vi "Update Log Status Values.vi"(1 "RT Data in":T1={"Device Ref"=18446744073709551615, "Waveforms"=[], "Channels"={"Command Chan Refs"=[], "Command Data Refs"=[], "Command Values"=[], "Status Chan Refs"=[], "Status Data Refs"=[], "Status Values"=[], "System Time"={"System Time"=timestamp(0 s since 1904-01-01), "Data Reference"=0, "Absolute Time Channel Data Ref"=0, "Get Date-Time Channel Data Ref"=0}, "Trigger Chan Refs"=[], "Trigger Data Refs"=[], "Trigger Values"=[]}, "Waveform Logs"=[], "Communication"={"Async Status"=refnum, "Wfm Comm Properties"={"WPL"={"Custom Queue Size"=1, "Use Custom Queue Size?"=FALSE}}, "Shutdown Event"=refnum, "Trigger Event"=refnum, "New File Event"=refnum, "Log Queues"=[], "Async VI Ref"=refnum}, "error"={"status"=FALSE, "code"=0, "source"=""}} {"Device Ref" format="%.0x"; "Channels"."Trigger Data Refs"."Data Reference" format="%.0x"; "Channels"."Trigger Chan Refs" format="%.0x"; "Channels"."System Time"."Get Date-Time Channel Data Ref" format="%.0x"; "Channels"."System Time"."Absolute Time Channel Data Ref" format="%.0x"; "Channels"."System Time"."Channel Data Reference" format="%.0x"; "Channels"."Status Data Refs"."Data Reference" format="%.0x"; "Channels"."Command Data Refs"."Data Reference" format="%.0x"; "Channels"."Status Chan Refs" format="%.0x"; "Channels"."Command Chan Refs" format="%.0x"; "Waveforms"."Waveform Ref in" format="%.0x"; "Waveform Logs"."Node ID" format="%.0x"; "Waveform Logs"."TDMS Error Code"."Data Ref" format="%.0x"; "Waveform Logs"."Missed Samples"."Data Ref" format="%.0x"; "Waveform Logs"."File Status"."Data Ref" format="%.0x"; "Waveform Logs"."Start New File"."Data Ref" format="%.0x"; "Waveform Logs"."Logging Enabled"."Data Ref" format="%.0x"; "Waveform Logs"."Stop Trigger"."Node Data Ref" format="%.0x"; "Waveform Logs"."Stop Trigger"."Node ID" format="%.0x"; "Waveform Logs"."Start Trigger"."Node Data Ref" format="%.0x"; "Waveform Logs"."Start Trigger"."Node ID" format="%.0x"}) -> (0 "RT Data out":T1={"Device Ref"=18446744073709551615, "Waveforms"=[], "Channels"={"Command Chan Refs"=[], "Command Data Refs"=[], "Command Values"=[], "Status Chan Refs"=[], "Status Data Refs"=[], "Status Values"=[], "System Time"={"System Time"=timestamp(0 s since 1904-01-01), "Data Reference"=0, "Absolute Time Channel Data Ref"=0, "Get Date-Time Channel Data Ref"=0}, "Trigger Chan Refs"=[], "Trigger Data Refs"=[], "Trigger Values"=[]}, "Waveform Logs"=[], "Communication"={"Async Status"=refnum, "Wfm Comm Properties"={"WPL"={"Custom Queue Size"=1, "Use Custom Queue Size?"=FALSE}}, "Shutdown Event"=refnum, "Trigger Event"=refnum, "New File Event"=refnum, "Log Queues"=[], "Async VI Ref"=refnum}, "error"={"status"=FALSE, "code"=0, "source"=""}} {"Device Ref" format="%.0x"; "Channels"."Trigger Data Refs"."Data Reference" format="%.0x"; "Channels"."Trigger Chan Refs" format="%.0x"; "Channels"."System Time"."Get Date-Time Channel Data Ref" format="%.0x"; "Channels"."System Time"."Absolute Time Channel Data Ref" format="%.0x"; "Channels"."System Time"."Channel Data Reference" format="%.0x"; "Channels"."Status Data Refs"."Data Reference" format="%.0x"; "Channels"."Command Data Refs"."Data Reference" format="%.0x"; "Channels"."Status Chan Refs" format="%.0x"; "Channels"."Command Chan Refs" format="%.0x"; "Waveforms"."Waveform Ref in" format="%.0x"; "Waveform Logs"."Node ID" format="%.0x"; "Waveform Logs"."TDMS Error Code"."Data Ref" format="%.0x"; "Waveform Logs"."Missed Samples"."Data Ref" format="%.0x"; "Waveform Logs"."File Status"."Data Ref" format="%.0x"; "Waveform Logs"."Start New File"."Data Ref" format="%.0x"; "Waveform Logs"."Logging Enabled"."Data Ref" format="%.0x"; "Waveform Logs"."Stop Trigger"."Node Data Ref" format="%.0x"; "Waveform Logs"."Stop Trigger"."Node ID" format="%.0x"; "Waveform Logs"."Start Trigger"."Node Data Ref" format="%.0x"; "Waveform Logs"."Start Trigger"."Node ID" format="%.0x"})   [LabVIEW 2015, in "Waveform Data Logger Engine.lvlib"]
uses:
  Waveform Data Logger Engine.lvlib
  Types/RT Data.ctl
  <vilib>/NI Veristand/Custom Device API/Custom Device Item Ref.ctl
  Types/Inline Waveform Info.ctl
  <vilib>/NI Veristand/Custom Device API/Waveform Data Reference.ctl
  Classes/Waveforms/Waveform Receive/Associated Log.ctl
  <vilib>/NI Veristand/Custom Device API/Custom Device Waveform DataType.ctl
  Types/Channels.ctl
  <vilib>/NI Veristand/Custom Device API/Block Data Reference.ctl
  <vilib>/NI Veristand/Custom Device API/Data Reference.ctl
  Types/System Time.ctl
  Types/Inline Waveform Log Info.ctl
  Classes/Log File Specifications/Waveform TDMS Log File Specification/Waveform TDMS Log File Specification.lvclass
  Classes/Triggers/Trigger/Trigger.lvclass
  Types/Inline Log Waveform.ctl
  Types/Trigger Settings.ctl
  Types/Log Status.ctl
  Types/Channel.ctl
  Types/Communication.ctl
  Types/Async Status.ctl
  Types/Async State.ctl
  <vilib>/NI Veristand/Custom Device Waveform API/Communication Properties.ctl
  Types/Trigger Event Data.ctl
  Types/Trigger Received.ctl
  Types/New File Event Data.ctl
  Types/Log Queues.ctl
  <vilib>/NI Veristand/Custom Device API/Custom Device API.lvlib
  Classes/Waveforms/Waveform Receive/Waveform Receive.lvclass
  <vilib>/NI Veristand/Custom Device Waveform API/NI_VS Custom Device Waveform API.lvlib
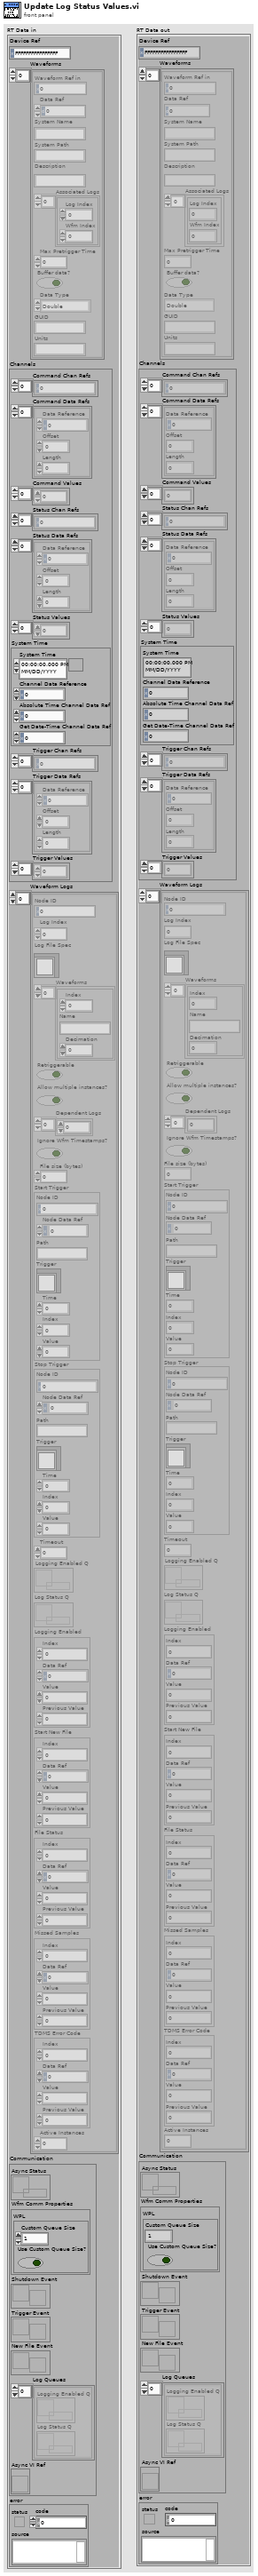
[diagram p1: front panel]
types:
  T1 = typedef "Waveform Data Logger Engine.lvlib/RT Data.ctl" = cluster{"Device Ref":T2, "Waveforms":T3[], "Channels":T7, "Waveform Logs":T11[], "Communication":T15, "error":errorcluster}
  T2 = typedef "Custom Device API.lvlib/Custom Device Item Ref.ctl" = u64
  T3 = typedef "Waveform Data Logger Engine.lvlib/Inline Waveform Info.ctl" = cluster{"Waveform Ref in":T2, "Data Ref":T4, "System Name":string, "System Path":string, "Description":string, "Associated Logs":T5[], "Max Pretrigger Time":dbl, "Buffer data?":bool, "Data Type":T6, "GUID":string, "Units":string}
  T4 = typedef "Custom Device API.lvlib/Waveform Data Reference.ctl" = i32
  T5 = typedef "Waveform Receive.lvclass/Associated Log.ctl" = cluster{"Log Index":i32, "Wfm Index":i32}
  T6 = typedef "Custom Device API.lvlib/Custom Device Waveform DataType.ctl" = enum16{"Double", "Complex Double"}
  T7 = typedef "Waveform Data Logger Engine.lvlib/Channels.ctl" = cluster{"Command Chan Refs":T2[], "Command Data Refs":T8[], "Command Values":dbl[], "Status Chan Refs":T2[], "Status Data Refs":T8[], "Status Values":dbl[], "System Time":T10, "Trigger Chan Refs":T2[], "Trigger Data Refs":T8[], "Trigger Values":dbl[]}
  T8 = typedef "Custom Device API.lvlib/Block Data Reference.ctl" = cluster{"Data Reference":T9, "Offset":u64, "Length":u64}
  T9 = typedef "Custom Device API.lvlib/Data Reference.ctl" = i32
  T10 = typedef "Waveform Data Logger Engine.lvlib/System Time.ctl" = cluster{"System Time":timestamp, "Data Reference":T9, "Absolute Time Channel Data Ref":T9, "Get Date-Time Channel Data Ref":T9}
  T11 = typedef "Waveform Data Logger Engine.lvlib/Inline Waveform Log Info.ctl" = cluster{"Node ID":T2, "Log Index":i32, "Log File Spec":refnum<class "Waveform TDMS Log File Specification.lvclass">, "Waveforms":T12[], "Retriggerable":bool, "Allow multiple instances?":bool, "Dependent Logs":i32[], "Ignore Wfm Timestamps?":bool, "File size (bytes)":i64, "Start Trigger":T13, "Stop Trigger":T13, "Timeout":dbl, "Logging Enabled Q":refnum<queue>, "Log Status Q":refnum<queue>, "Logging Enabled":T14, "Start New File":T14, "File Status":T14, "Missed Samples":T14, "TDMS Error Code":T14, "Active Instances":i32}
  T12 = typedef "Waveform Data Logger Engine.lvlib/Inline Log Waveform.ctl" = cluster{"Index":i32, "Name":string, "Decimation":u32}
  T13 = typedef "Waveform Data Logger Engine.lvlib/Trigger Settings.ctl" = cluster{"Node ID":T2, "Node Data Ref":i32, "Path":string, "Trigger":refnum<class "Trigger.lvclass">, "Time":dbl, "Index":i32, "Value":dbl}
  T14 = typedef "Waveform Data Logger Engine.lvlib/Channel.ctl" = cluster{"Index":i32, "Data Ref":T9, "Value":dbl, "Previous Value":dbl}
  T15 = typedef "Waveform Data Logger Engine.lvlib/Communication.ctl" = cluster{"Async Status":refnum<queue>, "Wfm Comm Properties":T16, "Shutdown Event":refnum<user-event>, "Trigger Event":refnum<user-event>, "New File Event":refnum<user-event>, "Log Queues":T17[], "Async VI Ref":refnum<vi>}
  T16 = typedef "NI_VS Custom Device Waveform API.lvlib/Communication Properties.ctl" = cluster{"WPL":cluster{"Custom Queue Size":i32, "Use Custom Queue Size?":bool}}
  T17 = typedef "Waveform Data Logger Engine.lvlib/Log Queues.ctl" = cluster{"Logging Enabled Q":refnum<queue>, "Log Status Q":refnum<queue>}
  T18 = typedef "Waveform Data Logger Engine.lvlib/Log Status.ctl" = cluster{"Open Instances":i32, "Active Instances":i32, "Missed Samples":u64, "Error Code":i32}
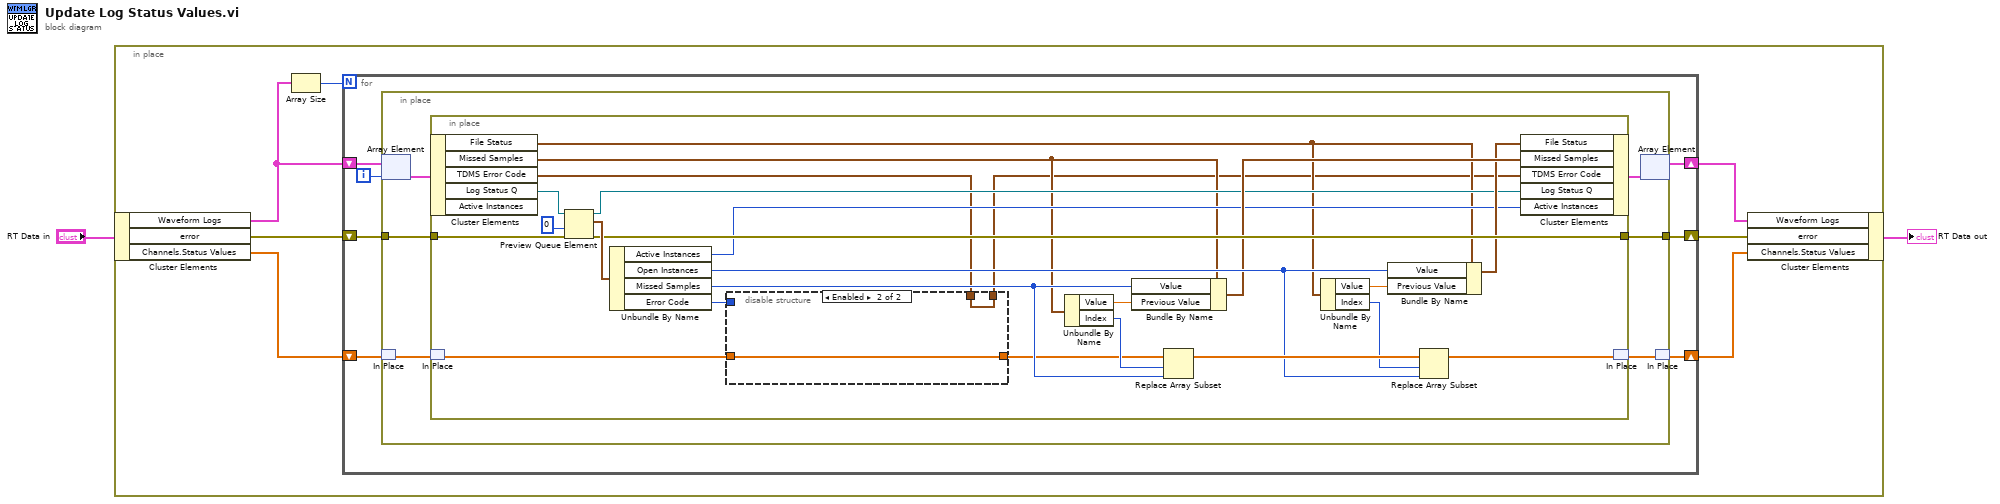
[diagram p0: block diagram]
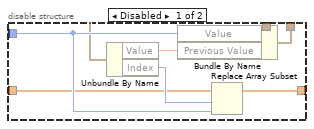
[diagram p2: hidden frame]
diagram:
  n1 = in-place {
    n2 = in-place-cluster #1("RT Data in") -> ("Waveform Logs"=w7:T11[], "error"=w9:errorcluster, "Channels.Status Values"=w4:dbl[])
    n3 = Array Size(array=w7) -> (size(s)=w8:i32)
    n4 = for {
      N: w8 -> [_]
      shift-right: [w12] -> w6
      shift-left: w9 -> [w16]
      shift-right: [w13] -> w5
      shift-left: w7 -> [w14]
      shift-right: [w10] -> w3
      shift-left: w4 -> [w11]
      i -> [w15]
      n5 = in-place {
        in-place-border: w16 -> [w22]
        in-place-border: [w21] -> w12
        n6 = in-place-array #2(w14, w15) -> (w18:T11)
        n7 = in-place-match #3(w11) -> (w20:dbl[])
        n8 = in-place {
          in-place-border: w22 -> [w44]
          in-place-border: [w43] -> w21
          n9 = in-place-cluster #4(w18) -> ("File Status"=w27:T14, "Missed Samples"=w30:T14, "TDMS Error Code"=w23:T14, "Log Status Q"=w34:refnum<queue>)  [unwired: 1 out]
          n10 = in-place-match #5(w20) -> (w41:dbl[])
          n11 = Preview Queue Element(queue=w34, timeout in ms (-1)=0, error in (no error)=w44) -> (queue out=w33:refnum<queue>, element=w45:T18, error out=w43:errorcluster)  [unwired: 1 out]
          n12 = Unbundle By Name(w45) -> ("Active Instances"=w32:i32, "Open Instances"=w39:i32, "Missed Samples"=w38:u64, "Error Code"=w26:i32)
          n13 = disable-structure shown="Enabled" {
            disable-tunnel: w26 -> [w51 _]
            disable-tunnel: [w50 w55] -> w25
            disable-tunnel: w23 -> [w49 w55]
            disable-tunnel: w41 -> [w48 w54]
            disable-tunnel: [w47 w54] -> w24
            frame Disabled {
              n14 = Unbundle By Name(w49) -> ("Value"=w53:dbl, "Index"=w52:i32)
              n15 = Bundle By Name(cluster=w49, "Value"=w51, "Previous Value"=w53) -> (w50:T14)
              n16 = Replace Array Subset(array=w48, new element=w51, index=w52) -> (w47:dbl[])
            }
            frame Enabled {
            }
          }
          n17 = Unbundle By Name(w30) -> ("Value"=w31:dbl, "Index"=w36:i32)
          n18 = Bundle By Name(cluster=w30, "Value"=w38, "Previous Value"=w31) -> (w37:T14)
          n19 = Replace Array Subset(array=w24, new element=w38, index=w36) -> (w42:dbl[])
          n20 = Unbundle By Name(w27) -> ("Value"=w29:dbl, "Index"=w28:i32)
          n21 = Bundle By Name(cluster=w27, "Value"=w39, "Previous Value"=w29) -> (w35:T14)
          n22 = Replace Array Subset(array=w42, new element=w39, index=w28) -> (w40:dbl[])
          n23 = in-place-cluster #4("File Status"=w35, "Missed Samples"=w37, "TDMS Error Code"=w25, "Log Status Q"=w33, "Active Instances"=w32) -> (w17:T11)
          n24 = in-place-match #5(w40) -> (w19:dbl[])
        }
        n25 = in-place-array #2(w17) -> (w13:T11[])  [unwired: 1 out]
        n26 = in-place-match #3(w19) -> (w10:dbl[])
      }
    }
    n27 = in-place-cluster #1("Waveform Logs"=w5, "error"=w6, "Channels.Status Values"=w3) -> (→"RT Data out":T1)
  }
